vi "generate file data from system.vi"(8 "error in":errorcluster, 11 "system":T1) -> (0 "error out":errorcluster, 3 "file information":T4)   [LabVIEW 2013, in "PLConfigurationSerializer.lvlib"]
uses:
  PLConfigurationSerializer.lvlib
  1_0_0_0 format.ctl
  system hierarchy.ctl
  target hierarchy.ctl
  engine hierarchy.ctl
  configuration database.ctl
  systems cluster.ctl
  system configuration/PL_System Configuration.lvclass
  targets cluster.ctl
  target configuration/PL_Target Configuration.lvclass
  engines cluster.ctl
  <vilib>/NI/Module Execution Interface/Engine Configuration/engine configuration.lvclass
  <vilib>/NI/Tag Bus Module Framework/module configuration/TBM module configuration.lvclass
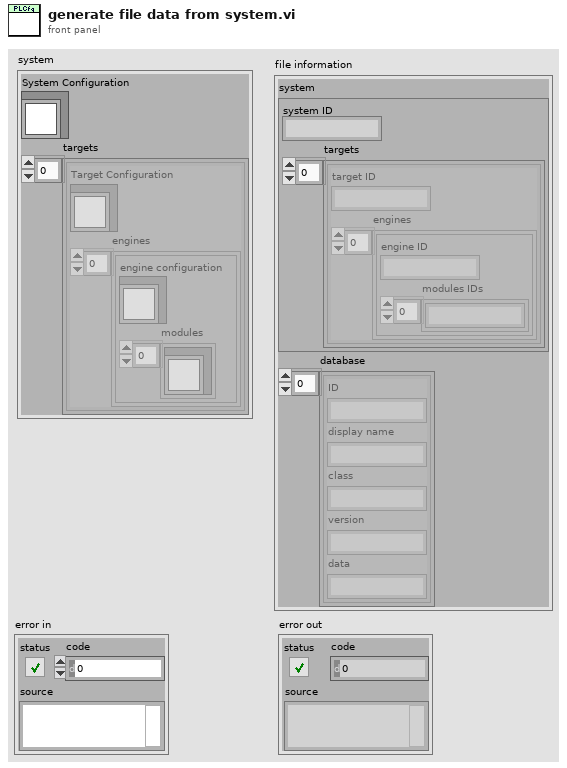
[diagram p1: front panel]
types:
  T1 = typedef "PLConfigurationSerializer.lvlib/systems cluster.ctl" = cluster{"System Configuration":refnum<class "PL_System Configuration.lvclass">, "targets":T2[]}
  T2 = typedef "PLConfigurationSerializer.lvlib/targets cluster.ctl" = cluster{"Target Configuration":refnum<class "PL_Target Configuration.lvclass">, "engines":T3[]}
  T3 = typedef "PLConfigurationSerializer.lvlib/engines cluster.ctl" = cluster{"engine configuration":refnum<class "engine configuration.lvclass">, "modules":refnum<class "TBM module configuration.lvclass">[]}
  T4 = typedef "PLConfigurationSerializer.lvlib/1_0_0_0 format.ctl" = cluster{"system":T5, "database":T8[]}
  T5 = typedef "PLConfigurationSerializer.lvlib/system hierarchy.ctl" = cluster{"system ID":string, "targets":T6[]}
  T6 = typedef "PLConfigurationSerializer.lvlib/target hierarchy.ctl" = cluster{"target ID":string, "engines":T7[]}
  T7 = typedef "PLConfigurationSerializer.lvlib/engine hierarchy.ctl" = cluster{"engine ID":string, "modules IDs":string[]}
  T8 = typedef "PLConfigurationSerializer.lvlib/configuration database.ctl" = cluster{"ID":string, "display name":string, "class":string, "version":string, "data":string}
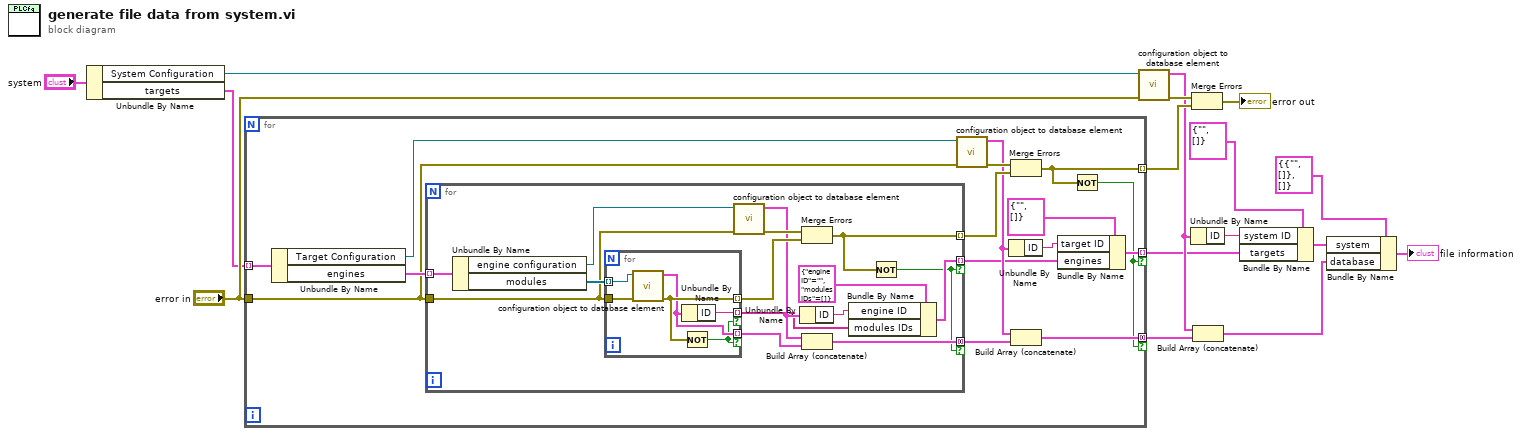
[diagram p0: block diagram]
diagram:
  n1 = Unbundle By Name("system") -> ("System Configuration"=w9:refnum<class "PL_System Configuration.lvclass">, "targets"=w13:T2[])
  n2 = for {
    tunnel: w13 -> [w31] mode=indexing
    tunnel: "error in" -> [w29]
    tunnel: [w25] -> w12 mode=concatenating if=w19
    tunnel: [w23] -> w11 mode=indexing
    tunnel: [w20] -> w2 mode=indexing if=w19
    n3 = Unbundle By Name(w31) -> ("Target Configuration"=w27:refnum<class "PL_Target Configuration.lvclass">, "engines"=w30:T3[])
    n4 = for {
      tunnel: w30 -> [w46] mode=indexing
      tunnel: w29 -> [w43]
      tunnel: [w40] -> w26 mode=concatenating if=w32
      tunnel: [w38] -> w28 mode=indexing
      tunnel: [w33] -> w18 mode=indexing if=w32
      n5 = Unbundle By Name(w46) -> ("engine configuration"=w42:refnum<class "engine configuration.lvclass">, "modules"=w45:refnum<class "TBM module configuration.lvclass">[])
      n6 = for {
        tunnel: w43 -> [w51]
        tunnel: w45 -> [w52] mode=indexing
        tunnel: [w49] -> w41 mode=indexing if=w47
        tunnel: [w50] -> w44 mode=indexing
        tunnel: [w48] -> w34 mode=indexing if=w47
        n7 = call "configuration object to database element.vi"("error in"=w51, "configuration in"=w52) -> ("error out"=w50:errorcluster, "database"=w49:T8)  [unwired: 8 in]
        n8 = Unbundle By Name(w49) -> ("ID"=w48:string)
        n9 = Not(x=w50) -> (.not. x?=w47:bool)
      }
      n10 = call "configuration object to database element.vi"("error in"=w43, "configuration in"=w42) -> ("error out"=w39:errorcluster, "database"=w37:T8)  [unwired: 8 in]
      n11 = Unbundle By Name(w37) -> ("ID"=w35:string)
      n12 = Merge Errors(w39, w44) -> (w38:errorcluster)
      n13 = Build Array (concatenate)(w37, w41) -> (w40:T8[])
      n14 = Bundle By Name(cluster=T7 {"engine ID"="", "modules IDs"=[]} ("engines cluster"), "engine ID"=w35, "modules IDs"=w34) -> (w33:T7)
      n15 = Not(x=w38) -> (.not. x?=w32:bool)
    }
    n16 = call "configuration object to database element.vi"("error in"=w29, "configuration in"=w27) -> ("error out"=w24:errorcluster, "database"=w22:T8)  [unwired: 8 in]
    n17 = Unbundle By Name(w22) -> ("ID"=w17:string)
    n18 = Merge Errors(w24, w28) -> (w23:errorcluster)
    n19 = Build Array (concatenate)(w22, w26) -> (w25:T8[])
    n20 = Bundle By Name(cluster=T6 {"target ID"="", "engines"=[]} ("targets cluster"), "target ID"=w17, "engines"=w18) -> (w20:T6)
    n21 = Not(x=w23) -> (.not. x?=w19:bool)
  }
  n22 = call "configuration object to database element.vi"("error in"="error in", "configuration in"=w9) -> ("error out"=w10:errorcluster, "database"=w5:T8)  [unwired: 8 in]
  n23 = Unbundle By Name(w5) -> ("ID"=w3:string)
  n24 = Merge Errors(w10, w11) -> (→"error out":errorcluster)
  n25 = Build Array (concatenate)(w5, w12) -> (w6:T8[])
  n26 = Bundle By Name(cluster=T5 {"system ID"="", "targets"=[]} ("system"), "system ID"=w3, "targets"=w2) -> (w1:T5)
  n27 = Bundle By Name(cluster=T4 {"system"={"system ID"="", "targets"=[]}, "database"=[]} ("1.0.0.0"), "system"=w1, "database"=w6) -> (→"file information":T4)
